vi "Wrap Value.vi"(7 "Max Index":i32, 11 "Value":i32) -> (3 "Wraped Value":i32)   [LabVIEW 2024]
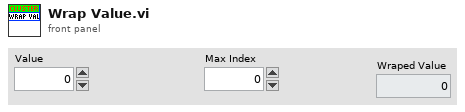
[diagram p1: front panel]
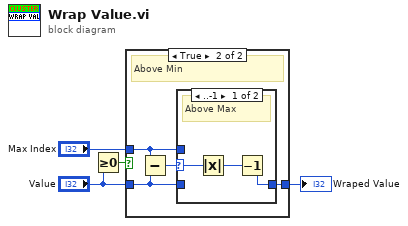
[diagram p0: block diagram]
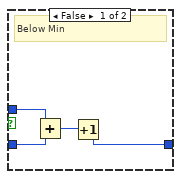
[diagram p2: hidden frame]
diagram:
  n1 = Greater Or Equal To 0?(x="Value") -> (x >= 0?=w2:bool)
  n2 = case shown="True" w2 {
    tunnel: "Max Index" -> [w8 w9]
    tunnel: "Value" -> [w7 w11]
    tunnel: [w5 w10] -> w1
    frame False {
      # "Below Min"
      n3 = Add(x=w8, y=w7) -> (x+y=w6:i32)
      n4 = Increment(x=w6) -> (x+1=w5:i32)
    }
    frame True {
      # "Above Min"
      n5 = Subtract(x=w9, y=w11) -> (x-y=w12:i32)
      n6 = case shown="..-1" w12 {
        selector: w12 -> [w15 _]
        tunnel: w11 -> [_ w16]
        tunnel: [w13 w16] -> w10
        tunnel: w9 -> [_ _]
        frame ..-1 {
          # "Above Max"
          n7 = Absolute Value(x=w15) -> (abs(x)=w14:i32)
          n8 = Decrement(x=w14) -> (x-1=w13:i32)
        }
        frame 0.. {
          # "Below Max"
        }
      }
    }
  }
  "Wraped Value" <- w1
